vi "ProcessJSONMulligans.vi"(8 "error in (no error)":errorcluster, 10 "JSON Array":string) -> (0 "error out":errorcluster, 1 "JSON Error string":string, 2 "Mulligans Requested":i32)   [LabVIEW 2013]
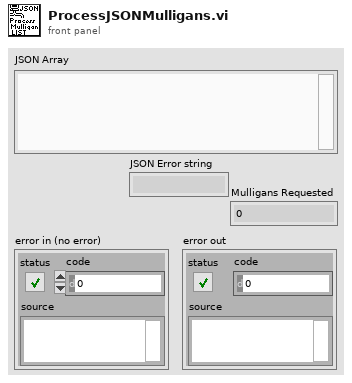
[diagram p1: front panel]
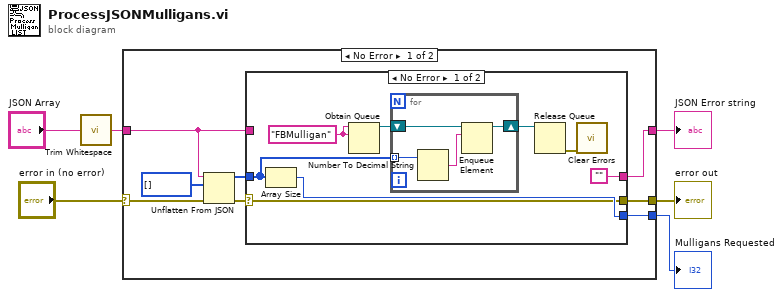
[diagram p0: block diagram]
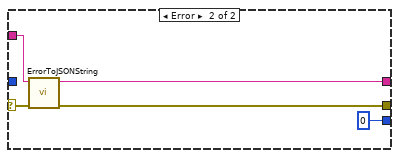
[diagram p2: hidden frame]
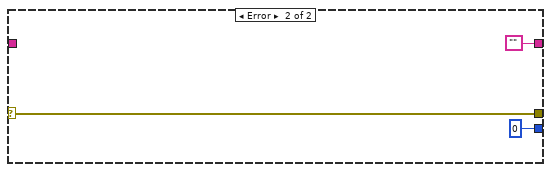
[diagram p3: hidden frame]
diagram:
  n1 = call <vilib>:"Trim Whitespace.vi"("string"="JSON Array") -> ("trimmed string"=w2:string)  [unwired: 1 in]
  n2 = case shown="No Error" "error in (no error)" {
    selector: "error in (no error)" -> [w13 w34]
    tunnel: w2 -> [w8 _]
    tunnel: [w9 w34] -> w6
    tunnel: [w12 0 ("offset past token")] -> w4
    tunnel: [w7 ""] -> w1
    frame No Error {
      n3 = Unflatten From JSON(JSON string=w8, type and defaults=i32[] [], error in (no error)=w13) -> (value=w11:i32[], error out=w10:errorcluster)  [unwired: 4 in]
      n4 = case shown="No Error" w10 {
        selector: w10 -> [w16 w31]
        tunnel: [w22 0] -> w12
        tunnel: w11 -> [w21 _]
        tunnel: [w16 w30] -> w9
        tunnel: w8 -> [_ w29]
        tunnel: ["" w28] -> w7
        frame No Error {
          w20 = "FBMulligan" ("name (unnamed)")
          n5 = Array Size(array=w21) -> (size(s)=w22:i32)
          n6 = Obtain Queue(name (unnamed)=w20, element data type=w20) -> (queue out=w19:refnum<queue>)  [unwired: 3 in, 2 out]
          n7 = for {
            tunnel: w21 -> [w26] mode=indexing
            shift-right: [w24] -> w17
            shift-left: w19 -> [w25]
            n8 = Number To Decimal String(number=w26) -> (decimal integer string=w23:string)  [unwired: 1 in]
            n9 = Enqueue Element(queue=w25, element=w23) -> (queue out=w24:refnum<queue>)  [unwired: 2 in, 2 out]
          }
          n10 = Release Queue(queue=w17) -> (error out=w18:errorcluster)  [unwired: 2 in, 2 out]
          n11 = call <vilib>:"Clear Errors.vi"("error in (no error)"=w18) -> ()  [unwired: 6 in, 1 out]
        }
        frame Error {
          n12 = call "ErrorToJSONString.vi"("error in (no error)"=w31, "problemJSON"=w29) -> ("error out"=w30:errorcluster, "JSON Error string"=w28:string)  [unwired: 8 in]
        }
      }
    }
    frame Error {
    }
  }
  "error out" <- w6
  "Mulligans Requested" <- w4
  "JSON Error string" <- w1
